vi "CompareVersion.vi"(11 "local file path out":path) -> (1 "NewVersion":string, 3 "FoundNew":bool)   [LabVIEW 2015]
uses:
  <vilib>/regexp/Match Regular Expression.xnode
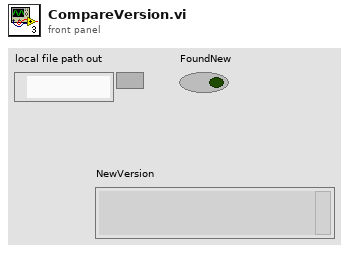
[diagram p1: front panel]
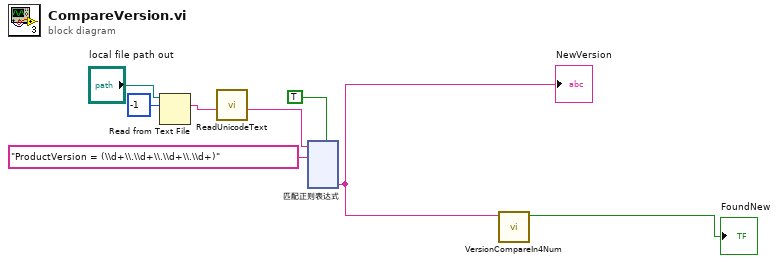
[diagram p0: block diagram]
diagram:
  n1 = Read from Text File(file (use dialog)="local file path out", count=-1 ("计数")) -> (text=w7:string)  [unwired: 2 in, 3 out]
  n2 = call "ReadUnicodeText.vi"("txtIn"=w7) -> ("result string"=w2:string)  [unwired: 9 in]
  n3 = xnode "匹配正则表达式"("输入字符串"=w2, "正则表达式"="ProductVersion = (\\d+\\.\\d+\\.\\d+\\.\\d+)", "多行？(F)"=TRUE) -> ("子匹配 1"=w1:string)  [unwired: 3 in, 5 out]
  "NewVersion" <- w1
  n4 = call "VersionCompareIn4Num.vi"("VersionOnWeb"=w1) -> ("realFoundNew"=→"FoundNew":bool)  [unwired: 10 in]
